vi "ParseSetConnectedDvr.vi"(8 "error in (no error)":errorcluster, 11 "body":variant) -> (0 "error out":errorcluster, 3 "connected":T1)   [LabVIEW 2017, in "ServerComm.lvlib"]
uses:
  <vilib>/addons/InsightCM/Devices/Shared/Common/ServerComm/ServerComm.lvlib
  <vilib>/addons/InsightCM/Devices/Shared/Common/ServerComm/controls/ConnectedStatusDvr.ctl
  <vilib>/addons/InsightCM/Devices/Shared/Common/ServerComm/controls/ConnectionStatus.ctl
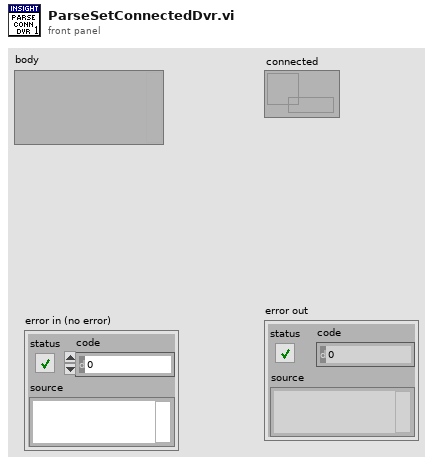
[diagram p1: front panel]
types:
  T1 = typedef "ServerComm.lvlib/ConnectedStatusDvr.ctl" = refnum<data-value>
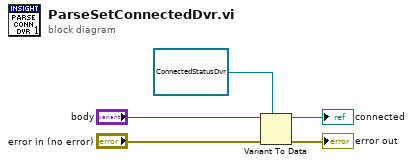
[diagram p0: block diagram]
diagram:
  w1 = T1 refnum items=["Offline", "NotAuthorized", "Online"] ("connected")
  n1 = Variant To Data(error in="error in (no error)", type=w1, Variant="body") -> (data=→"connected":T1, error out=→"error out":errorcluster)
